vi "Button Pressed.vi"(0 "reference in":refnum<class "Panel.lvclass">, 5 "error in (no error)":errorcluster) -> (14 "reference out":refnum<class "Panel.lvclass">, 19 "error out":errorcluster)   [LabVIEW 2013, in "Panel.lvclass"]
uses:
  Panel.lvclass
  Command_class/Command.lvclass
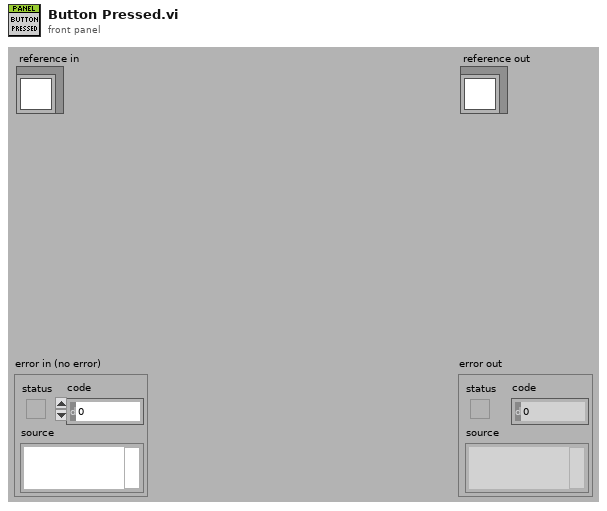
[diagram p1: front panel]
types:
  T1 = typedef "Panel.lvclass/ObjectAttributes.ctl" = cluster{"Command.lvclass":refnum<class "Command.lvclass">}
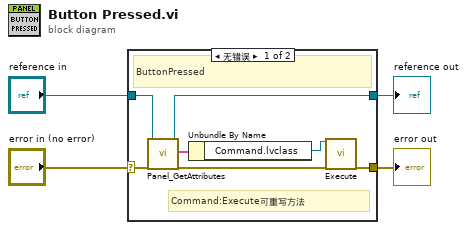
[diagram p0: block diagram]
diagram:
  n1 = case shown="无错误" "error in (no error)" {
    selector: "error in (no error)" -> [w11 w13]
    tunnel: [w5 w13] -> w3
    tunnel: [w10 w12] -> w1
    tunnel: "reference in" -> [w8 w12]
    frame No Error {
      # "Command:Execute可重写方法"
      # "ButtonPressed"
      n2 = call "Panel_GetAttributes.vi"("reference in"=w8, "error in (no error)"=w11) -> ("reference out"=w10:refnum<class "Panel.lvclass">, "attributes"=w9:T1, "error out"=w6:errorcluster)  [unwired: 14 in, 1 out]
      n3 = Unbundle By Name(w9) -> ("Command.lvclass"=w7:refnum<class "Command.lvclass">)
      n4 = call-dynamic "Execute.vi"("reference in"=w7, "error in (no error)"=w6) -> ("error out"=w5:errorcluster)  [unwired: 16 in, 1 out]
    }
    frame Error {
    }
  }
  "error out" <- w3
  "reference out" <- w1
